vi "CRYAna Perceptual Rub&Buzz.vi"(6 "TSR params":T1 {"Sweep Time" format="%.2f"; "Amplit" format="%.2f"; "FStop" format="%.2f"; "FStart" format="%.2f"; "FSamp" format="%.2f"; "Tsamp" format="%.2f"; "NHarm" format="%.2f"; "MStart" format="%.2f"; "MStop" format="%.2f"; "NOffset" format="%.2f"}, 7 "Harmonic Infor":T2={"Cycles"=[200.0, 190.0, 180.0, 170.0, 160.0, 150.0, 140.0, 132.0, 125.0, 118.0, 112.0, 106.0, 100.0, 95.0, 90.0, 85.0, 80.0, 75.0, 71.0, 67.0, 63.0, 60.0, 56.0, 53.0, 50.0, 48.0, 45.0, 43.0, 40.0, 38.0, 36.0, 34.0, 32.0, 30.0, 28.0, 27.0, 25.0, 24.0, 23.0, 22.0, 20.0, 19.0, 18.0, 17.0, 16.0, 15.0, 14.0, 14.0, 13.0, 12.0, 12.0, 11.0, 10.0, 10.0, 9.0, 9.0, 8.0, 8.0, 8.0, 7.0, 7.0, 6.0, 6.0, 6.0, 6.0, 6.0, 6.0, 6.0, 6.0, 6.0, 6.0, 6.0, 6.0, 6.0, 8.0, 8.0, 8.0, 8.0, 8.0, 8.0, 8.0, 8.0], "Frequency"=[20000.0, 19000.0, 18000.0, 17000.0, 16000.0, 15000.0, 14000.0, 13199.999809265137, 12500.0, 11800.000190734863, 11199.999809265137, 10600.000381469727, 10000.0, 9500.0, 9000.0, 8500.0, 8000.0, 7500.0, 7099.999904632568, 6699.999809265137, 6300.000190734863, 6000.0, 5599.999904632568, 5300.000190734863, 5000.0, 4750.0, 4500.0, 4250.0, 4000.0, 3750.0, 3549.999952316284, 3349.9999046325684, 3150.0000953674316, 3000.0, 2799.999952316284, 2650.0000953674316, 2500.0, 2359.999895095825, 2240.000009536743, 2119.999885559082, 2000.0, 1900.0, 1800.0, 1700.0, 1600.0, 1500.0, 1400.0, 1319.9999809265137, 1250.0, 1180.0000190734863, 1119.9999809265137, 1060.0000381469727, 1000.0, 950.0, 900.0, 850.0, 800.0, 750.0, 709.9999904632568, 669.9999809265137, 630.0000190734863, 600.0, 559.9999904632568, 530.0000190734863, 500.0, 475.0, 450.0, 425.0, 400.0, 375.0, 354.9999952316284, 334.99999046325684, 315.00000953674316, 300.0, 250.0, 200.0, 160.0, 125.0, 100.0, 80.0, 63.00000190734863, 50.0], "Amplitude"=[0.5, 0.5, 0.5, 0.5, 0.5, 0.5, 0.5, 0.5, 0.5, 0.5, 0.5, 0.5, 0.5, 0.5, 0.5, 0.5, 0.5, 0.5, 0.5, 0.5, 0.5, 0.5, 0.5, 0.5, 0.5, 0.5, 0.5, 0.5, 0.5, 0.5, 0.5, 0.5, 0.5, 0.5, 0.5, 0.5, 0.5, 0.5, 0.5, 0.5, 0.5, 0.5, 0.5, 0.5, 0.5, 0.5, 0.5, 0.5, 0.5, 0.5, 0.5, 0.5, 0.5, 0.5, 0.5, 0.5, 0.5, 0.5, 0.5, 0.5, 0.5, 0.5, 0.5, 0.5, 0.5, 0.5, 0.5, 0.5, 0.5, 0.5, 0.5, 0.5, 0.5, 0.5, 0.5, 0.5, 0.5, 0.5, 0.5, 0.5, 0.5, 0.5], "samples"=[441, 441, 441, 441, 441, 441, 441, 441, 441, 441, 441, 441, 441, 441, 441, 441, 441, 441, 441, 441, 441, 441, 441, 441, 441, 446, 441, 446, 441, 447, 447, 447, 448, 441, 441, 450, 441, 448, 453, 458, 441, 441, 441, 441, 441, 441, 441, 467, 459, 448, 473, 458, 441, 464, 441, 467, 441, 470, 497, 461, 490, 441, 472, 499, 530, 557, 588, 622, 662, 705, 746, 790, 840, 882, 1411, 1764, 2205, 2823, 3528, 4410, 5600, 7055], "Fs"=44100.0, "window"=7, "discard cycles"=1.0} {"discard cycles" min=1.0}, 8 "Harmonic Track In":T3(array[cluster]), 9 "Response":dbl[](array[numeric])=array[67013 elements], 10 "Stimulus":dbl[](array[numeric])=array[64855 elements], 11 "Algorithm":u16=2) -> (0 "Harmonic Track Out":T3(array[cluster]))   [LabVIEW 2013]
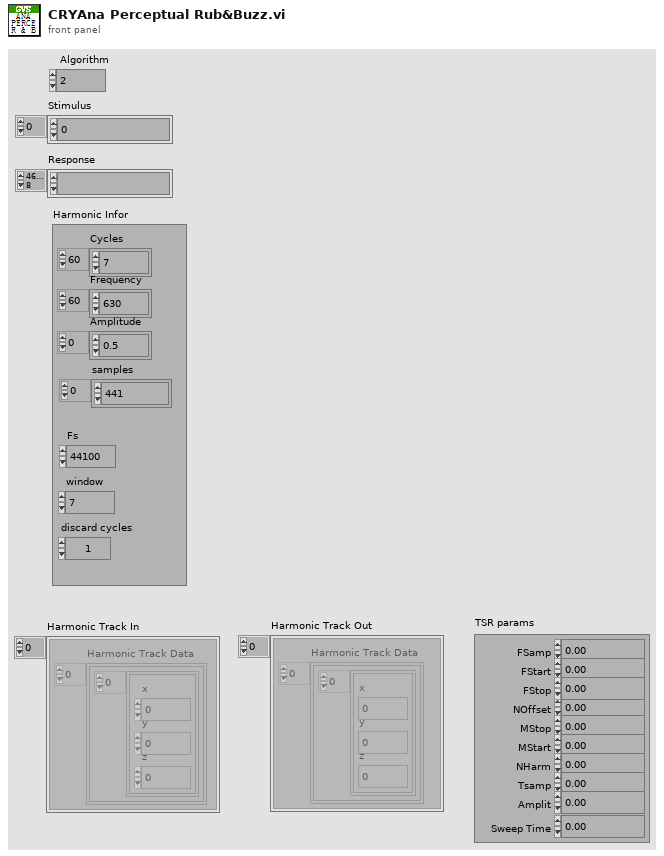
[diagram p1: front panel]
types:
  T1 = cluster{"FSamp":dbl, "FStart":dbl, "FStop":dbl, "NOffset":dbl, "MStop":dbl, "MStart":dbl, "NHarm":dbl, "Tsamp":dbl, "Amplit":dbl, "Sweep Time":dbl}
  T2 = cluster{"Cycles":dbl[], "Frequency":dbl[], "Amplitude":dbl[], "samples":i32[], "Fs":dbl, "window":u16, "discard cycles":dbl}
  T3 = cluster{"Harmonic Track Data":cluster{cluster{"x":dbl, "y":dbl, "z":dbl}[]}[]}[]
  T4 = cluster{"element":dbl, "element":dbl, "element":dbl}[]
  T5 = cluster{cluster{"element":dbl, "element":dbl, "element":dbl}[]}
  T6 = cluster{cluster{"element":dbl, "element":dbl, "element":dbl}[]}[]
  T7 = cluster{"Harmonic Track Data":cluster{cluster{"element":dbl, "element":dbl, "element":dbl}[]}[]}[]
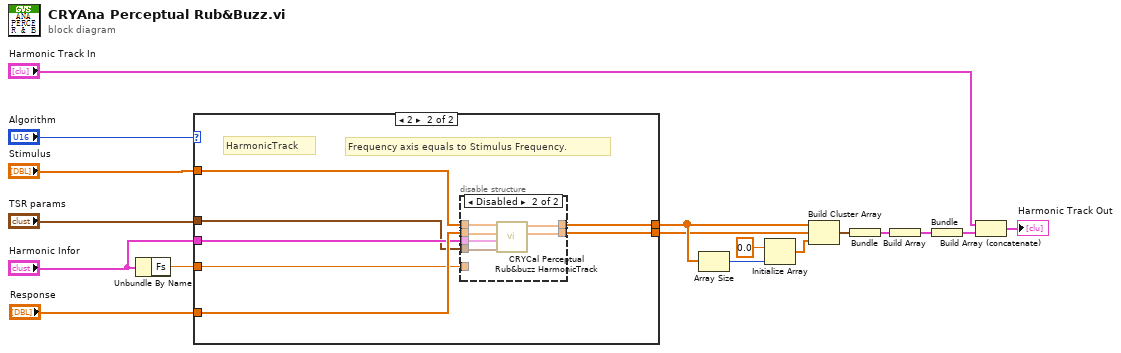
[diagram p0: block diagram]
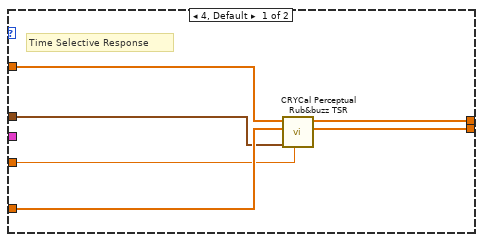
[diagram p2: hidden frame]
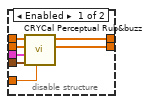
[diagram p3: hidden frame]
diagram:
  n1 = Unbundle By Name("Harmonic Infor") -> ("Fs"=w15:dbl)
  n2 = case shown="2" "Algorithm" {
    tunnel: w15 -> [w20 w25]
    tunnel: "Stimulus" -> [w23 w30]
    tunnel: "Response" -> [w22 w29]
    tunnel: [w19 w28] -> w10
    tunnel: [w18 w27] -> w9
    tunnel: "TSR params" -> [w21 w24]
    tunnel: "Harmonic Infor" -> [_ w26]
    frame 4, Default {
      # "Time Selective Response"
      n3 = call "CRYCal Perceptual Rub&buzz TSR.vi"("Fs"=w20, "TSR params"=w21, "Response"=w22, "Stimulus"=w23) -> ("EHS + NL"=w18:dbl[], "Frequency"=w19:dbl[])  [unwired: 6 in]
    }
    frame 2 {
      # "Frequency axis equals to Stimulus Frequency."
      # "HarmonicTrack"
      n4 = disable-structure shown="Disabled" {
        disable-tunnel: w30 -> [w37 w43]
        disable-tunnel: w29 -> [w36 w42]
        disable-tunnel: [w35 w39] -> w28
        disable-tunnel: [w34 w38] -> w27
        disable-tunnel: w26 -> [w33 w41]
        disable-tunnel: w25 -> [w32 _]
        disable-tunnel: w24 -> [w31 w40]
        frame Enabled {
          n5 = call "CRYCal Perceptual Rub&buzz.vi"("Fs"=w32, "TSR params"=w31, "Harmonic Infor"=w33, "Response"=w36, "Stimulus"=w37) -> ("EHS + NL"=w34:dbl[], "Frequency"=w35:dbl[])  [unwired: 5 in]
        }
        frame Disabled {
          n6 = call "CRYCal Perceptual Rub&buzz HarmonicTrack.vi"("TSR params"=w40, "Harmonic Infor"=w41, "Response"=w42, "Stimulus"=w43) -> ("EHS + NL"=w38:dbl[], "Frequency"=w39:dbl[])  [unwired: 6 in]
        }
      }
    }
  }
  n7 = Array Size(array=w10) -> (size(s)=w6:i32)
  n8 = Initialize Array(0.0 ("element"), w6) -> (w5:dbl[])
  n9 = Build Cluster Array(w10, w9, w5) -> (w2:T4)
  n10 = Bundle(w2) -> (w4:T5)  [unwired: 1 in]
  n11 = Build Array(w4) -> (w3:T6)
  n12 = Bundle(w3) -> (w16:cluster{cluster{cluster[]}[]})  [unwired: 1 in]
  n13 = Build Array (concatenate)("Harmonic Track In", w16) -> (→"Harmonic Track Out":T7)
